vi "dfd_X Equal Y (Scalar).vi"(0 "x":dbl, 3 "y":dbl, 4 "esp":dbl=1e-12) -> (6 "x = y?":bool)   [LabVIEW 2017, in "NI_DigFilterLicensed.lvlib"]
uses:
  <vilib>/addons/Digital Filter Design/NI_DigFilterLicensed.lvlib
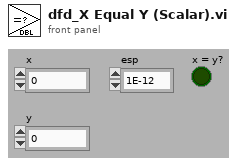
[diagram p1: front panel]
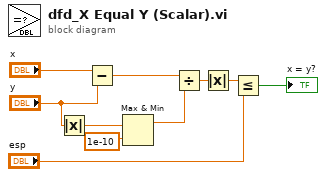
[diagram p0: block diagram]
diagram:
  n1 = Absolute Value(x="y") -> (abs(x)=w4:dbl)
  n2 = Subtract(x="x", y="y") -> (x-y=w8:dbl)
  n3 = Max & Min(x=w4, y=1e-10) -> (max(x,y)=w2:dbl)  [unwired: 1 out]
  n4 = Divide(x=w8, y=w2) -> (x/y=w9:dbl)
  n5 = Absolute Value(x=w9) -> (abs(x)=w10:dbl)
  n6 = Less Or Equal?(x=w10, y="esp") -> (x <= y?=→"x = y?":bool)
